vi "Create Deformation Sensor File.vi"   [LabVIEW 2019]
uses:
  <vilib>/Utility/miscctls.llb/LVDateTimeRec.ctl
  <vilib>/Utility/file.llb/Read Delimited Spreadsheet (string).vi
types:
  T1 = cluster{"Sensor Name":string, "Sensor Info":cluster{"Manufacturer":string, "Model":string, "Serial Number":string}, "Last Cal Info":cluster{"Last Calibration Date":dbl, "Calibrator":string, "Cal Duration":i32}, "Voltage Range":cluster{"High Limit":dbl, "Low Limit":dbl}, "EGU Range":cluster{"High Limit":dbl, "Low Limit":dbl}, "Units":string, "Calibration Type":enum16{"Calibrate Analog", "Compare Analog Calibration"}, "EGU List":dbl[], "Voltage List":dbl[], "Coefficients":dbl[], "Order":i32, "Algorithm":enum32{"SVD", "Givens", "Givens2", "Householder", "LU Decomposition", "Cholesky"}, "Max Error % of Full Scale":dbl, "Max Mean Squared Error":dbl, "Use Error %":bool, "Use MSE":bool, "Allow Manual Entry":bool, "Max Stability Error":dbl, "Max Error % of Reading":dbl, "Use Error % of Reading":bool}[]
  T2 = typedef "LVDateTimeRec.ctl" = cluster{"fractional second":dbl, "second":i32, "minute":i32, "hour":i32, "day of month":i32, "month":i32, "year":i32, "day of week":i32, "day of year":i32, "DST":i32}
  T3 = cluster{"Sensor Name":string, "Sensor Info":cluster{"Manufacturer":string, "Model":string, "Serial Number":string}, "Last Cal Info":cluster{"Last Calibration Date":dbl, "Calibrator":string, "Cal Duration":i32}, "Voltage Range":cluster{"High Limit":dbl, "Low Limit":dbl}, "EGU Range":cluster{"High Limit":dbl, "Low Limit":dbl}, "Units":string, "Calibration Type":enum16{"Calibrate Analog", "Compare Analog Calibration"}, "EGU List":dbl[], "Voltage List":dbl[], "Coefficients":dbl[], "Order":i32, "Algorithm":enum32{"SVD", "Givens", "Givens2", "Householder", "LU Decomposition", "Cholesky"}, "Max Error % of Full Scale":dbl, "Max Mean Squared Error":dbl, "Use Error %":bool, "Use MSE":bool, "Allow Manual Entry":bool, "Max Stability Error":dbl, "Max Error % of Reading":dbl, "Use Error % of Reading":bool}
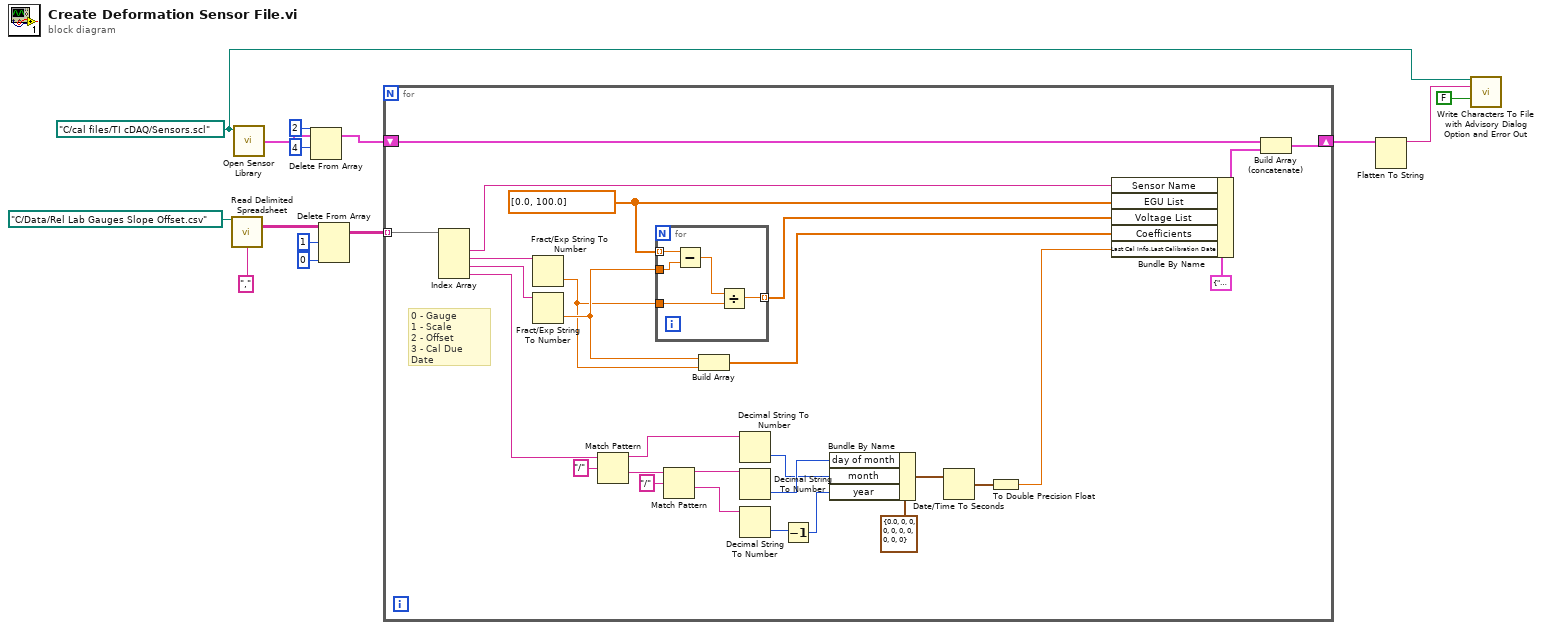
[diagram p0: block diagram]
diagram:
  w6 = path "C:/cal files/TI cDAQ/Sensors.scl" ("Sensor Library Path")
  n1 = call-poly <vilib>:"Read Delimited Spreadsheet.vi"("file path (dialog if empty)"=path "C:/Data/Rel Lab Gauges Slope Offset.csv", "delimiter (\\t)"="," ("delimiter (\\t)")) -> ("all rows"=w12:string[][])  [unwired: 8 in, 5 out]
  n2 = call "Open Sensor Library.vi"("Sensor Library Path"=w6) -> ("Sensors Info"=w4:T1)  [unwired: 4 in, 2 out]
  n3 = Delete From Array(array=w4, length=4, index=2) -> (array with subset deleted=w1:T1)  [unwired: 1 out]
  n4 = Delete From Array(array=w12, length=1, index (row)=0) -> (array with subset deleted=w9:string[][])  [unwired: 1 in, 1 out]
  n5 = for {
    shift-right: [w40] -> w5
    shift-left: w1 -> [w41]
    tunnel: w9 -> [w42] mode=indexing
    w34 = dbl[] [0.0, 100.0] ("EGU List")
    # "0 - Gauge\n1 - Scale\n2 - Offset\n3 - Cal Due Date"
    n6 = Index Array(array=w42) -> (element #1=w37:string, element #2=w36:string, element #3=w35:string, element #4=w19:string)  [unwired: 4 in]
    n7 = Fract/Exp String To Number(string=w36) -> (number=w31:dbl)  [unwired: 3 in, 1 out]
    n8 = Fract/Exp String To Number(string=w35) -> (number=w32:dbl)  [unwired: 3 in, 1 out]
    n9 = Match Pattern(string=w19, regular expression="/") -> (before substring=w24:string, after substring=w22:string)  [unwired: 1 in, 2 out]
    n10 = for {
      tunnel: w34 -> [w47] mode=indexing
      tunnel: [w45] -> w33 mode=indexing
      tunnel: w32 -> [w46]
      tunnel: w31 -> [w43]
      n11 = Subtract(x=w47, y=w46) -> (x-y=w44:dbl)
      n12 = Divide(x=w44, y=w43) -> (x/y=w45:dbl)
    }
    n13 = Match Pattern(string=w22, regular expression="/") -> (before substring=w26:string, after substring=w28:string)  [unwired: 1 in, 2 out]
    n14 = Build Array(w32, w31) -> (w30:dbl[])
    n15 = Decimal String To Number(string=w24) -> (number=w25:i32)  [unwired: 2 in, 1 out]
    n16 = Decimal String To Number(string=w26) -> (number=w27:i32)  [unwired: 2 in, 1 out]
    n17 = Decimal String To Number(string=w28) -> (number=w18:i32)  [unwired: 2 in, 1 out]
    n18 = Decrement(x=w18) -> (x-1=w17:i32)
    n19 = Bundle By Name(cluster=T2 {"fractional second"=0.0, "second"=0, "minute"=0, "hour"=0, "day of month"=0, "month"=0, "year"=0, "day of week"=0, "day of year"=0, "DST"=0} ("date time rec"), "day of month"=w27, "month"=w25, "year"=w17) -> (w29:T2)
    n20 = Date/Time To Seconds(2:w29) -> (0:w16:timestamp)  [unwired: 1 in]
    n21 = To Double Precision Float(number=w16) -> (double precision float=w15:dbl)
    n22 = Bundle By Name(cluster=T3 {"Sensor Name"="", "Sensor Info"={"Manufacturer"="", "Model"="", "Serial Number"=""}, "Last Cal Info"={"Last Calibration Date"=0.0, "Calibrator"="", "Cal Duration"=0}, "Voltage Range"={"High Limit"=0.0, "Low Limit"=0.0}, "EGU Range"={"High Limit"=0.0, "Low Limit"=0.0}, "Units"="", "Calibration Type"=enum."Calibrate Analog", "EGU List"=[], "Voltage List"=[], "Coefficients"=[], "Order"=0, "Algorithm"=enum."SVD", "Max Error % of Full Scale"=0.0, "Max Mean Squared Error"=0.0, "Use Error %"=FALSE, "Use MSE"=FALSE, "Allow Manual Entry"=FALSE, "Max Stability Error"=0.0, "Max Error % of Reading"=0.0, "Use Error % of Reading"=FALSE} ("Sensor Description"), "Sensor Name"=w37, "EGU List"=w34, "Voltage List"=w33, "Coefficients"=w30, "Last Cal Info.Last Calibration Date"=w15) -> (w38:T3)
    n23 = Build Array (concatenate)(w41, w38) -> (w40:T1)
  }
  n24 = Flatten To String(anything=w5) -> (data string=w8:string)  [unwired: 3 in, 2 out]
  n25 = call "Write Characters To File with Advisory Dialog Option and Error Out.vi"("file path (dialog if empty)"=w6, "character string"=w8, "advisory dialog? (display:T)"=FALSE) -> ()  [unwired: 11 in, 2 out]
